vi "Zero_Wheels.vi"(2 "Init":i32, 3 "Encoder_In":i32, 4 "Re_Init":bool, 5 "Zero_Trigger":bool) -> (0 "Encoder_Out":i32, 1 "Reset_Trigger":bool)   [LabVIEW 2018]
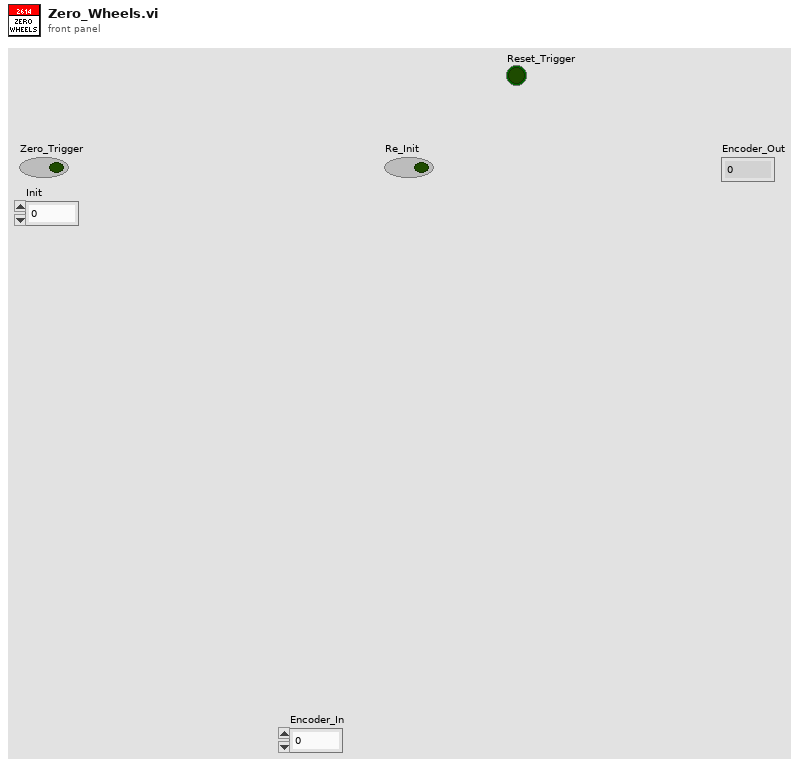
[diagram p1: front panel]
types:
  T1 = enum16{"Wait_For_Offset", "Grab_Offset", "Subtract_Offset", "Feed_New_Value"}
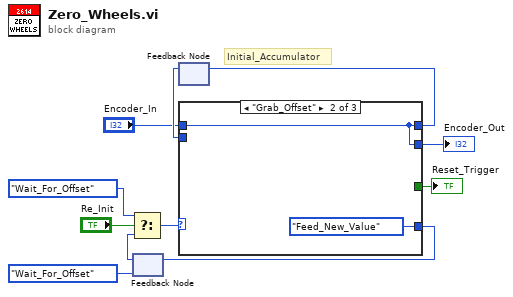
[diagram p0: block diagram]
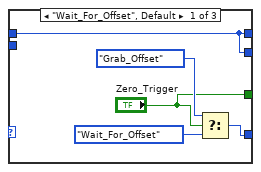
[diagram p2: hidden frame]
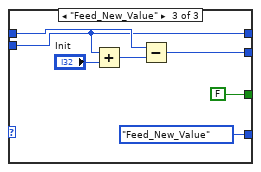
[diagram p3: hidden frame]
diagram:
  # "Initial_Accumulator"
  n1 = feedback #1(T1."Wait_For_Offset") -> (w5:T1)
  n2 = Select(t=T1."Wait_For_Offset", s="Re_Init", f=w5) -> (s? t:f=w4:T1)
  n3 = feedback #2() -> (w10:i32)  [unwired: 1 in]
  n4 = case shown="\"Grab_Offset\"" w4 {
    tunnel: [w16 T1."Feed_New_Value" T1."Feed_New_Value"] -> w8
    tunnel: [w13 w17 w23] -> w9
    tunnel: "Encoder_In" -> [w13 w17 w24]
    tunnel: w10 -> [_ _ w23]
    tunnel: [w13 w17 w21] -> w7
    tunnel: ["Zero_Trigger" _ FALSE] -> w1
    frame "Wait_For_Offset", Default {
      n5 = Select(t=T1."Grab_Offset", s="Zero_Trigger", f=T1."Wait_For_Offset") -> (s? t:f=w16:T1)
    }
    frame "Grab_Offset" {
    }
    frame "Feed_New_Value" {
      n6 = Add(x=w23, y="Init") -> (x+y=w22:i32)
      n7 = Subtract(x=w24, y=w22) -> (x-y=w21:i32)
    }
  }
  "Encoder_Out" <- w7
  "Reset_Trigger" <- w1
  n8 = feedback-in #1(w8) -> ()
  n9 = feedback-in #2(w9) -> ()
